vi "Config-Sweep-SMU Pulse.vi"(7 "base (V or A)":dbl format="%^.4e", 8 "error in (no error)":errorcluster, 9 "width (sec)":dbl=0.01 format="%.4f", 10 "period (sec)":dbl=0.1 format="%.4f", 11 "VISA session":refnum<visa-resource-name>) -> (0 "error out":errorcluster, 3 "VISA resource name out":refnum<visa-resource-name>)   [LabVIEW 2016, in "Agilent 415X Series.lvlib"]
doc: "This VI configures pulse parameters of a SMU if its mode is set to VPLUSE or IPULSE.\n\n** This VI should be used only when one of the SMUs has its mode set to VPULSE or IPULSE."
uses:
  Agilent 415X Series.lvlib
panel:
  # "This VI should be used only\nwhen one of the SMUs is in\nVPULSE or IPULSE mode."
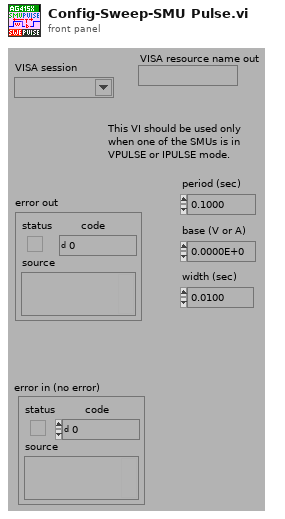
[diagram p1: front panel]
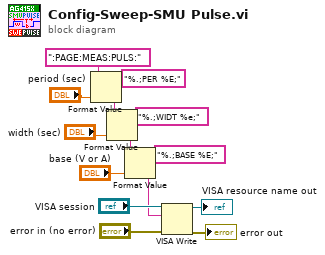
[diagram p0: block diagram]
diagram:
  n1 = Format Value(string ("")=":PAGE:MEAS:PULS:", format string="%.;PER %E;", value (0)="period (sec)") -> (output string=w11:string)
  n2 = Format Value(string ("")=w11, format string="%.;WIDT %e;", value (0)="width (sec)") -> (output string=w3:string)
  n3 = Format Value(string ("")=w3, format string="%.;BASE %E;", value (0)="base (V or A)") -> (output string=w2:string)
  n4 = VISA Write(VISA resource name="VISA session", write buffer=w2, error in (no error)="error in (no error)") -> (VISA resource name out=→"VISA resource name out":refnum<visa-resource-name>, error out=→"error out":errorcluster)  [unwired: 1 out]
